vi "Read Floating Number Format.vi"(8 "error in (no error)":errorcluster, 11 "Serializer.openg-ini in":refnum<class "Serializer.openg-ini.lvclass">) -> (0 "error out":errorcluster, 2 "Floating Number Format":string, 3 "Serializer.openg-ini out":refnum<class "Serializer.openg-ini.lvclass">)   [LabVIEW 2019, in "OpenSerializer.OpenG-ini.lvlib" / "Serializer.openg-ini.lvclass"]
uses:
  Serializer.openg-ini.lvclass
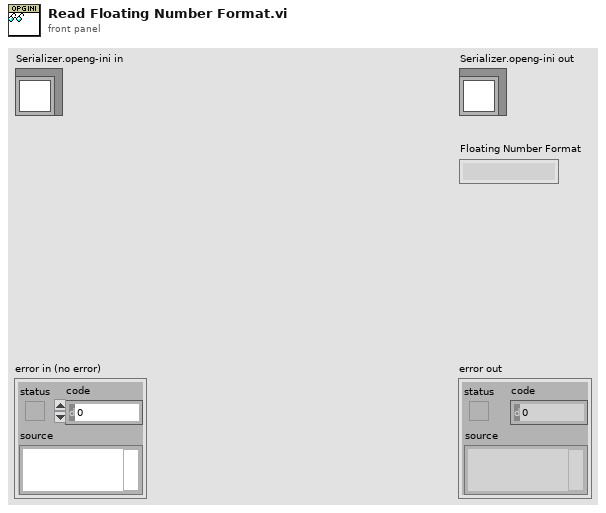
[diagram p1: front panel]
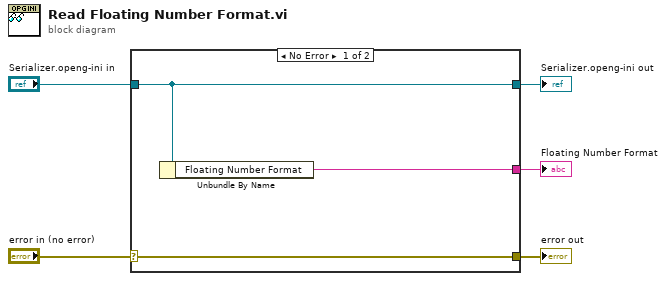
[diagram p0: block diagram]
diagram:
  n1 = case shown="No Error" "error in (no error)" {
    selector: "error in (no error)" -> [w8 w9]
    tunnel: [w8 w9] -> w4
    tunnel: [w7 w10] -> w2
    tunnel: "Serializer.openg-ini in" -> [w7 w10]
    tunnel: [w6 _] -> w1
    frame No Error {
      n2 = Unbundle By Name(w7) -> ("Floating Number Format"=w6:string)
    }
    frame Error {
    }
  }
  "error out" <- w4
  "Serializer.openg-ini out" <- w2
  "Floating Number Format" <- w1
